vi "Create Network Stream Listener.vi"(6 "Buffer Size":i32=4096, 11 "Name":string) -> (3 "Network Stream Listener":refnum<class "Network Stream Listener.lvclass">)   [LabVIEW 2020, in "Network Stream Listener.lvclass"]
doc: "Use this method to configure a Network Stream Listener for use."
uses:
  <vilib>/NI/Actors/Network Endpoint Actors/Protocols/Network Stream Strategy/Netowrk Stream Listener/Network Stream Listener.lvclass
  C:/Program Files (x86)/National Instruments/LabVIEW 2020/vi.lib/NI/Actors/Network Endpoint Actors/Protocols/Network Stream Strategy/Network Stream/Network Stream.lvclass
  <vilib>/NI/Actors/Network Endpoint Actors/Protocols/Network Stream Strategy/Network Stream/Network Stream.lvclass/Network Stream.ctl
  <vilib>/NI/Actors/Network Endpoint Actors/Protocols/Network Stream Strategy/Network Stream/Network Stream.lvclass
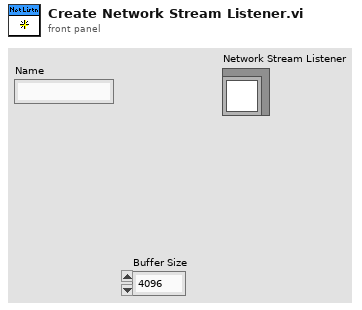
[diagram p1: front panel]
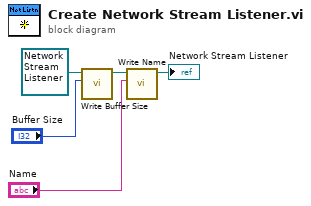
[diagram p0: block diagram]
diagram:
  n1 = call <vilib>:"Write Buffer Size.vi"("Buffer Size"="Buffer Size", "Network Stream in"=refnum<class "Network Stream Listener.lvclass"> refnum ("Network Stream Listener in")) -> ("Network Stream out"=w4:refnum<class "Network Stream Listener.lvclass">)  [unwired: 9 in]
  n2 = call <vilib>:"Write Name.vi"("Name"="Name", "Network Stream in"=w4) -> ("Network Stream out"=→"Network Stream Listener":refnum<class "Network Stream Listener.lvclass">)  [unwired: 9 in]
